vi "Return_chk.vi"(8 "에러 입력(에러 없음)":errorcluster, 11 "VISA 참조 번호 입력":refnum<visa-resource-name>) -> (0 "에러 출력":errorcluster, 2 "불리언":bool, 3 "VISA 참조 번호 출력":refnum<visa-resource-name>)   [LabVIEW 2023]
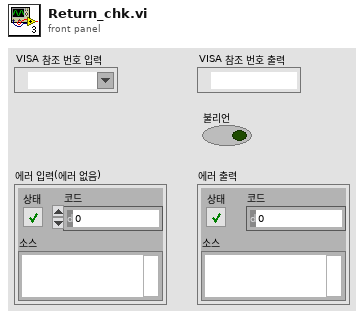
[diagram p1: front panel]
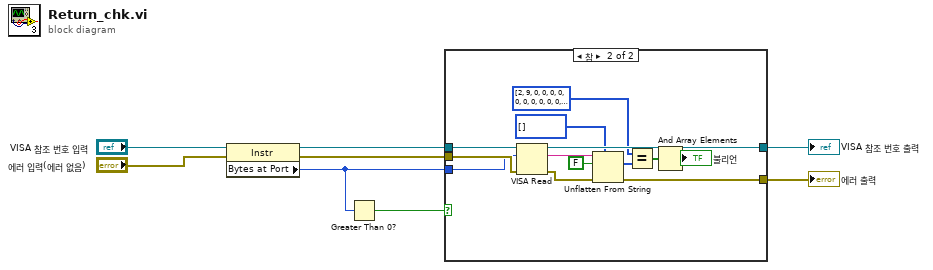
[diagram p0: block diagram]
diagram:
  n1 = property class="Instr"(reference="VISA 참조 번호 입력", error in="에러 입력(에러 없음)") -> (reference out=w5:refnum<visa-resource-name>, error out=w6:errorcluster, "Bytes at Port"=w2:u32)
  n2 = Greater Than 0?(x=w2) -> (x > 0?=w1:bool)
  n3 = case shown="참" w1 {
    tunnel: [w9 w23] -> w8
    tunnel: [w10 w22] -> w7
    tunnel: w6 -> [w10 w13]
    tunnel: w2 -> [_ w12]
    tunnel: w5 -> [w9 w11]
    frame False {
    }
    frame True {
      n4 = VISA Read(VISA resource name=w11, byte count=w12, error in (no error)=w13) -> (VISA resource name out=w23:refnum<visa-resource-name>, read buffer=w14:string, error out=w15:errorcluster)  [unwired: 1 out]
      n5 = Unflatten From String(type=i16[] [], binary string=w14, data includes array or string size? (T)=FALSE ("데이터가 배열 또는 문자열 크기를 포함? (참)"), error in (no error)=w15) -> (value=w18:i16[], error out=w22:errorcluster)  [unwired: 1 in, 1 out]
      n6 = Equal?(x=i16[] [2, 9, 0, 0, 0, 0, 0, 0, 0, 0, 0, 0, 3], y=w18) -> (x = y?=w20:bool[])
      n7 = And Array Elements(Boolean array=w20) -> (logical AND=→"불리언":bool)
    }
  }
  "VISA 참조 번호 출력" <- w8
  "에러 출력" <- w7
